vi "Graphics-Nice Histogram.vi"(0 "XYGraph":refnum<vi>, 5 "X-axis":refnum<vi>, 7 "Array":dbl[](array[numeric]), 11 "integer":bool) -> ()   [LabVIEW 2020]
uses:
  <vilib>/Analysis/polynomials.llb/Unique Numbers and Multiplicity (DBL).vi
  <vilib>/Analysis/NI_AALPro.lvlib
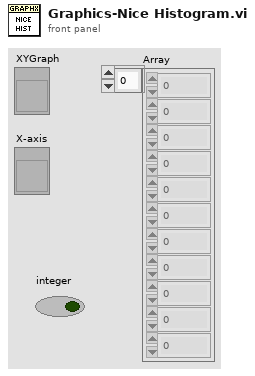
[diagram p1: front panel]
types:
  T1 = cluster{dbl, dbl, "inclusion":enum32{"lower", "upper", "both", "neither"}}
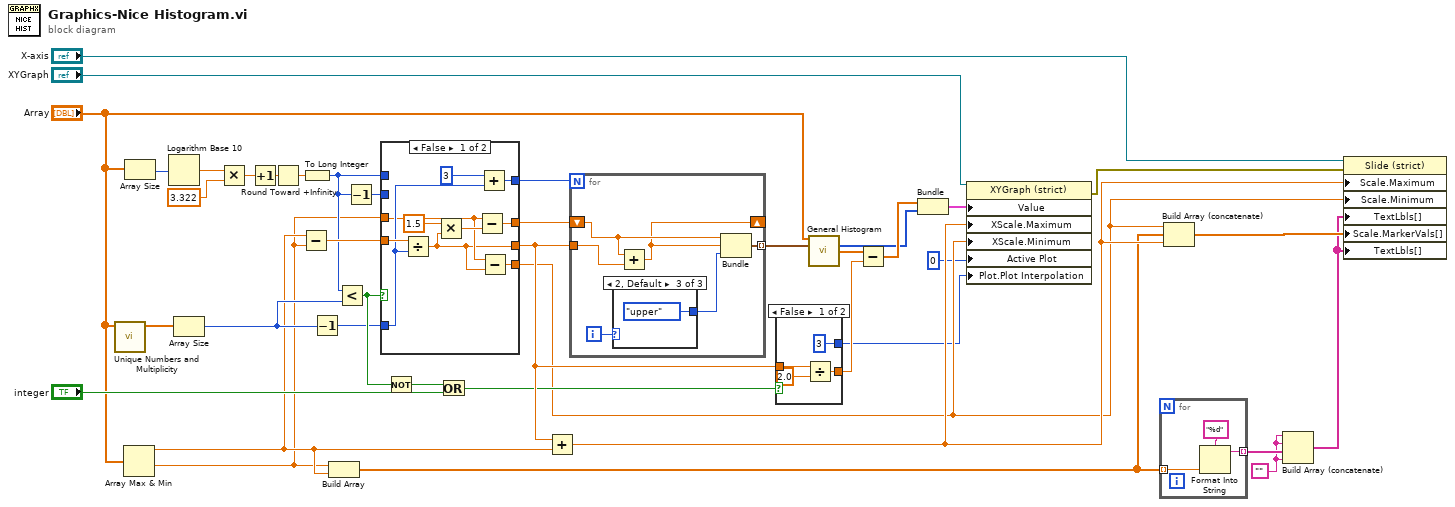
[diagram p0: block diagram]
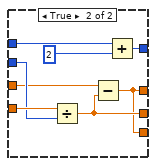
[diagram p2: hidden frame]
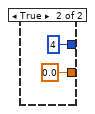
[diagram p3: hidden frame]
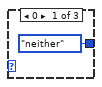
[diagram p4: hidden frame]
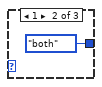
[diagram p5: hidden frame]
diagram:
  w19 = ""
  n1 = call-poly <vilib>:"Unique Numbers and Multiplicity.vi"("Numbers"="Array") -> ("Unique Numbers"=w16:dbl[])  [unwired: 8 in, 2 out]
  n2 = Array Max & Min(array="Array") -> (max value=w10:dbl, min value=w6:dbl)  [unwired: 2 out]
  n3 = Array Size(array="Array") -> (size(s)=w40:i32)
  n4 = Logarithm Base 10(1:w40) -> (0:w39:dbl)
  n5 = Array Size(array=w16) -> (size(s)=w13:i32)
  n6 = Multiply(x=w39, y=3.322) -> (x*y=w37:dbl)
  n7 = Increment(x=w37) -> (x+1=w35:dbl)
  n8 = Round Toward +Infinity(x=w35) -> (ceil(x): smallest int >= x=w34:dbl)
  n9 = Subtract(x=w10, y=w6) -> (x-y=w36:dbl)
  n10 = To Long Integer(number=w34) -> (32bit integer=w9:i32)
  n11 = Decrement(x=w13) -> (x-1=w7:i32)
  n12 = Build Array(w6, w10) -> (w21:dbl[])
  n13 = Less?(x=w9, y=w13) -> (x < y?=w12:bool)
  n14 = Decrement(x=w9) -> (x-1=w11:i32)
  n15 = case shown="False" w12 {
    tunnel: w36 -> [w50 w58]
    tunnel: [w42 w52] -> w27
    tunnel: w11 -> [_ w54]
    tunnel: w6 -> [w43 w53]
    tunnel: w9 -> [_ w56]
    tunnel: [w48 w55] -> w8
    tunnel: w7 -> [w47 _]
    tunnel: [w49 w51] -> w4
    tunnel: [w41 w51] -> w5
    frame False {
      n16 = Divide(x=w50, y=w47) -> (x/y=w42:dbl)
      n17 = Multiply(x=1.5, y=w42) -> (x*y=w45:dbl)
      n18 = Subtract(x=w43, y=w45) -> (x-y=w49:dbl)
      n19 = Add(x=3, y=w47) -> (x+y=w48:i32)
      n20 = Subtract(x=w43, y=w42) -> (x-y=w41:dbl)
    }
    frame True {
      n21 = Divide(x=w58, y=w54) -> (x/y=w52:dbl)
      n22 = Subtract(x=w53, y=w52) -> (x-y=w51:dbl)
      n23 = Add(x=w56, y=2) -> (x+y=w55:i32)
    }
  }
  n24 = Not(x=w12) -> (.not. x?=w14:bool)
  n25 = Or(x=w14, y="integer") -> (x .or. y?=w15:bool)
  n26 = Add(x=w27, y=w10) -> (x+y=w22:dbl)
  n27 = for {
    N: w8 -> [_]
    tunnel: w27 -> [w63]
    shift-right: [w62] -> _
    shift-left: w4 -> [w64]
    tunnel: [w61] -> w33 mode=indexing
    i -> [w60]
    n28 = case shown="2, Default" w60 {
      tunnel: [enum32{"lower", "upper", "both", "neither"}."neither" ("inclusion") enum32{"lower", "upper", "both", "neither"}."both" ("inclusion") enum32{"lower", "upper", "both", "neither"}."upper" ("inclusion")] -> w59
      frame 0 {
      }
      frame 1 {
      }
      frame 2, Default {
      }
    }
    n29 = Add(x=w64, y=w63) -> (x+y=w62:dbl)
    n30 = Bundle(w64, w62, "inclusion"=w59) -> (w61:T1)  [unwired: 1 in]
  }
  n31 = case shown="False" w15 {
    tunnel: w27 -> [w71 _]
    tunnel: [w69 0.0] -> w26
    tunnel: [u8 3 ("Plot.Plot Interpolation") u8 4 ("Plot.Plot Interpolation")] -> w1
    frame False {
      n32 = Divide(x=w71, y=2.0) -> (x/y=w69:dbl)
    }
    frame True {
    }
  }
  n33 = call <vilib>:"General Histogram.vi"("X"="Array", "Bins"=w33) -> ("Histogram"=w24:i32[], "Axis"=w28:dbl[])  [unwired: 9 in, 3 out]
  n34 = Subtract(x=w28, y=w26) -> (x-y=w25:dbl[])
  n35 = Bundle(w25, "Histogram"=w24) -> (w23:cluster{dbl[], "Histogram":i32[]})  [unwired: 1 in]
  n36 = property class="XYGraph (strict)"(reference="XYGraph", "Value"=w23, "XScale.Maximum"=w22, "XScale.Minimum"=w5, "Active Plot"=u32 0, "Plot.Plot Interpolation"=w1) -> (error out=w30:errorcluster)  [unwired: 1 in, 1 out]
  n37 = for {
    tunnel: w21 -> [w75] mode=indexing
    tunnel: [w74] -> w20 mode=indexing
    n38 = Format Into String(format string="%d", w75) -> (resulting string=w74:string)  [unwired: 2 in, 1 out]
  }
  n39 = Build Array (concatenate)(w5, w21, w22) -> (w29:dbl[])
  n40 = Build Array (concatenate)(w19, w19, w20, w19) -> (w3:string[])
  n41 = property class="Slide (strict)"(reference="X-axis", error in=w30, "Scale.Maximum"=w22, "Scale.Minimum"=w5, "TextLbls[]"=w3, "Scale.MarkerVals[]"=w29, "TextLbls[]"=w3) -> ()  [unwired: 2 out]
